vi "Ping_Dead.vi"(0 "ModelNumber":string, 1 "error in":errorcluster caption="错误输入（无错误）") -> (2 "Acess":bool, 3 "standard output":string caption="标准输出", 4 "error out":errorcluster caption="错误输出")   [LabVIEW 2013]
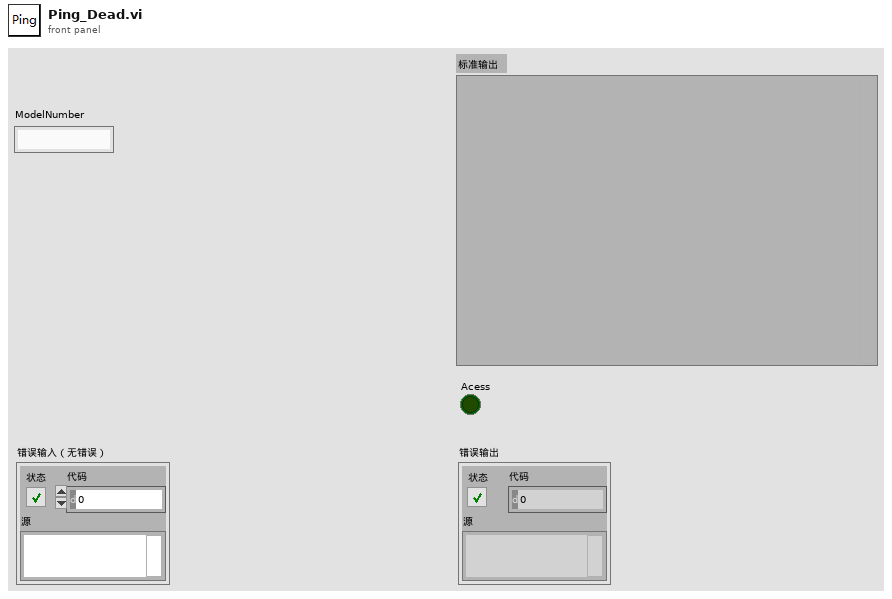
[diagram p1: front panel]
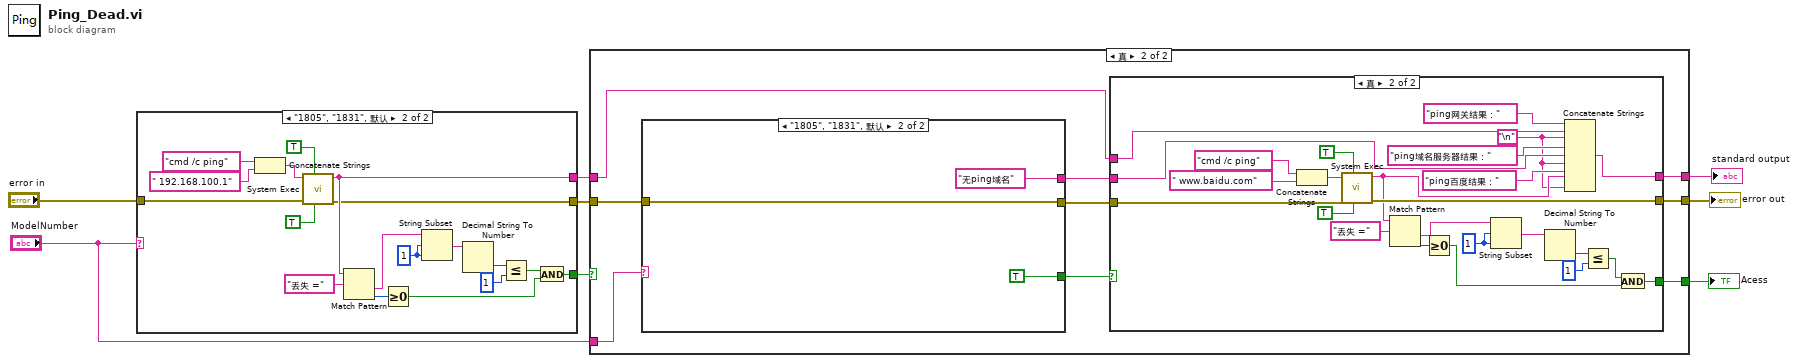
[diagram p0: block diagram]
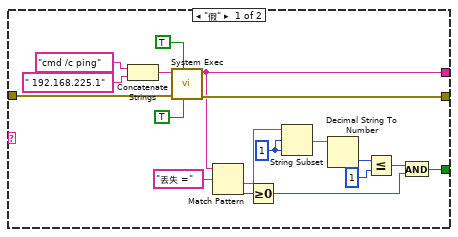
[diagram p2: hidden frame]
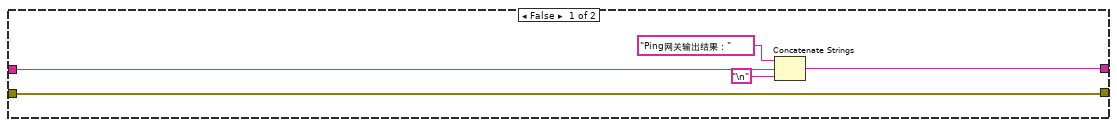
[diagram p3: hidden frame]
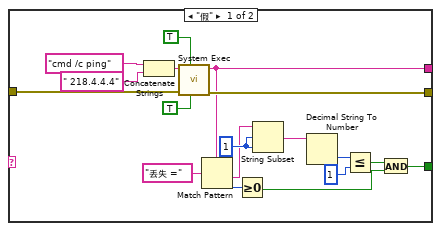
[diagram p4: hidden frame]
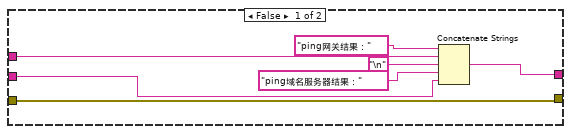
[diagram p5: hidden frame]
diagram:
  n1 = case shown="\"1805\", \"1831\", 默认" "ModelNumber" {
    tunnel: "error in" -> [w26 w29]
    tunnel: [w13 w28] -> w5
    tunnel: [w12 w27] -> w4
    tunnel: [w11 w30] -> w2
    frame "假" {
      w19 = 1
      n2 = Concatenate Strings("cmd /c ping" ("command line"), " 192.168.225.1" ("Adress")) -> (w23:string)
      n3 = call <vilib>:"System Exec.vi"("run minimized? (F)"=TRUE, "wait until completion? (T)"=TRUE ("run minimized? (F)"), "error in (no error)"=w26, "command line"=w23) -> ("error out"=w13:errorcluster, "standard output"=w11:string)  [unwired: 4 in, 2 out]
      n4 = Match Pattern(string=w11, regular expression="丢失 =" ("正则表达式")) -> (after substring=w18:string, offset past match=w17:i32)  [unwired: 1 in, 2 out]
      n5 = Greater Or Equal To 0?(x=w17) -> (x >= 0?=w14:bool)
      n6 = String Subset(string=w18, offset (0)=w19, length (rest)=w19) -> (substring=w20:string)
      n7 = Decimal String To Number(string=w20) -> (number=w21:i32)  [unwired: 2 in, 1 out]
      n8 = Less Or Equal?(x=w21, y=1) -> (x <= y?=w15:bool)
      n9 = And(x=w15, y=w14) -> (x .and. y?=w12:bool)
    }
    frame "1805", "1831", Default {
      w38 = 1
      n10 = Concatenate Strings("cmd /c ping" ("command line"), " 192.168.100.1" ("Adress")) -> (w42:string)
      n11 = call <vilib>:"System Exec.vi"("run minimized? (F)"=TRUE, "wait until completion? (T)"=TRUE ("run minimized? (F)"), "error in (no error)"=w29, "command line"=w42) -> ("error out"=w28:errorcluster, "standard output"=w30:string)  [unwired: 4 in, 2 out]
      n12 = Match Pattern(string=w30, regular expression="丢失 =" ("正则表达式")) -> (after substring=w37:string, offset past match=w36:i32)  [unwired: 1 in, 2 out]
      n13 = Greater Or Equal To 0?(x=w36) -> (x >= 0?=w33:bool)
      n14 = String Subset(string=w37, offset (0)=w38, length (rest)=w38) -> (substring=w39:string)
      n15 = Decimal String To Number(string=w39) -> (number=w40:i32)  [unwired: 2 in, 1 out]
      n16 = Less Or Equal?(x=w40, y=1) -> (x <= y?=w34:bool)
      n17 = And(x=w34, y=w33) -> (x .and. y?=w27:bool)
    }
  }
  n18 = case shown="真" w4 {
    tunnel: [_ w58] -> w8
    tunnel: [w49 w57] -> w7
    tunnel: w5 -> [w49 w56]
    tunnel: [w48 w54] -> w3
    tunnel: w2 -> [w46 w52]
    tunnel: "ModelNumber" -> [_ w50]
    frame False {
      n19 = Concatenate Strings("Ping网关输出结果：", w46, "\n") -> (w48:string)
    }
    frame True {
      n20 = case shown="\"1805\", \"1831\", 默认" w50 {
        tunnel: w56 -> [w74 w79]
        tunnel: [w72 w79] -> w55
        tunnel: [w63 TRUE ("run minimized? (F)")] -> w53
        tunnel: [w62 "无ping域名" ("standard output")] -> w51
        frame "假" {
          w67 = 1
          n21 = Concatenate Strings("cmd /c ping" ("command line"), " 218.4.4.4" ("Adress")) -> (w73:string)
          n22 = call <vilib>:"System Exec.vi"("run minimized? (F)"=TRUE, "wait until completion? (T)"=TRUE ("run minimized? (F)"), "error in (no error)"=w74, "command line"=w73) -> ("error out"=w72:errorcluster, "standard output"=w62:string)  [unwired: 4 in, 2 out]
          n23 = Match Pattern(string=w62, regular expression="丢失 =" ("正则表达式")) -> (after substring=w61:string, offset past match=w68:i32)  [unwired: 1 in, 2 out]
          n24 = Greater Or Equal To 0?(x=w68) -> (x >= 0?=w71:bool)
          n25 = String Subset(string=w61, offset (0)=w67, length (rest)=w67) -> (substring=w66:string)
          n26 = Decimal String To Number(string=w66) -> (number=w65:i32)  [unwired: 2 in, 1 out]
          n27 = Less Or Equal?(x=w65, y=1) -> (x <= y?=w70:bool)
          n28 = And(x=w70, y=w71) -> (x .and. y?=w63:bool)
        }
        frame "1805", "1831", Default {
        }
      }
      n29 = case shown="真" w53 {
        tunnel: [_ w101] -> w58
        tunnel: [w80 w100] -> w57
        tunnel: w55 -> [w80 w96]
        tunnel: [w81 w88] -> w54
        tunnel: w52 -> [w85 w94]
        tunnel: w51 -> [w82 w92]
        frame False {
          n30 = Concatenate Strings("ping网关结果：" ("command line"), w85, "\n", "ping域名服务器结果：" ("command line"), w82) -> (w81:string)
        }
        frame True {
          w89 = "\n"
          w107 = 1
          n31 = Concatenate Strings("cmd /c ping" ("command line"), " www.baidu.com" ("Adress")) -> (w99:string)
          n32 = call <vilib>:"System Exec.vi"("run minimized? (F)"=TRUE, "wait until completion? (T)"=TRUE ("run minimized? (F)"), "error in (no error)"=w96, "command line"=w99) -> ("error out"=w100:errorcluster, "standard output"=w90:string)  [unwired: 4 in, 2 out]
          n33 = Match Pattern(string=w90, regular expression="丢失 =" ("正则表达式")) -> (after substring=w108:string, offset past match=w109:i32)  [unwired: 1 in, 2 out]
          n34 = Greater Or Equal To 0?(x=w109) -> (x >= 0?=w102:bool)
          n35 = String Subset(string=w108, offset (0)=w107, length (rest)=w107) -> (substring=w106:string)
          n36 = Decimal String To Number(string=w106) -> (number=w105:i32)  [unwired: 2 in, 1 out]
          n37 = Concatenate Strings("ping网关结果：" ("command line"), w94, w89, "ping域名服务器结果：" ("command line"), w92, w89, "ping百度结果：" ("command line"), w90, w89) -> (w88:string)
          n38 = Less Or Equal?(x=w105, y=1) -> (x <= y?=w103:bool)
          n39 = And(x=w103, y=w102) -> (x .and. y?=w101:bool)
        }
      }
    }
  }
  "error out" <- w7
  "Acess" <- w8
  "standard output" <- w3
